vi "DAT Example.vi"() -> ()   [LabVIEW 2013]
panel:
  in  "wavenames (.Vx, etc)":string[](array[string])=["time", "temp", "Bfield", "X0", "Y0", "X1", "Y1", "X2", "Y2", "X3", "Y3", "X4", "Y4", "X5", "Y5"]
  in  "number4":dbl=7.0
  in  "number3":dbl=5.0
  in  "number2":dbl=3.0
  in  "number1":dbl
  out "plot2":cluster{"X":dbl[], "Y":dbl[]}[](graph)
  out "plot1":cluster{"X":dbl[], "Y":dbl[]}[](graph)
  out "plot0":cluster{"X":dbl[], "Y":dbl[]}[](graph)
  in  "Notes":string="date and time are AUTOMATICALLY saved!\nwrite your experiment notes here"
  in  "path":path=path "C:/"
  in  "filename":string="datatest"
  # "- set path to folder\n- set base filename\n   (up to 999,999 files with same base name \n    an be written in one folder)\n- type some comments"
  # "you usually display your data as a XY\ngraphs or charts:"
  # "give everything you are saving a name,\nor else you will become confused!"
  # "combine all of your data using \"build  array\" function\n\nEach entry represents one data point at a partiular time"
  # "\"numbers\" can be\n saved too:"
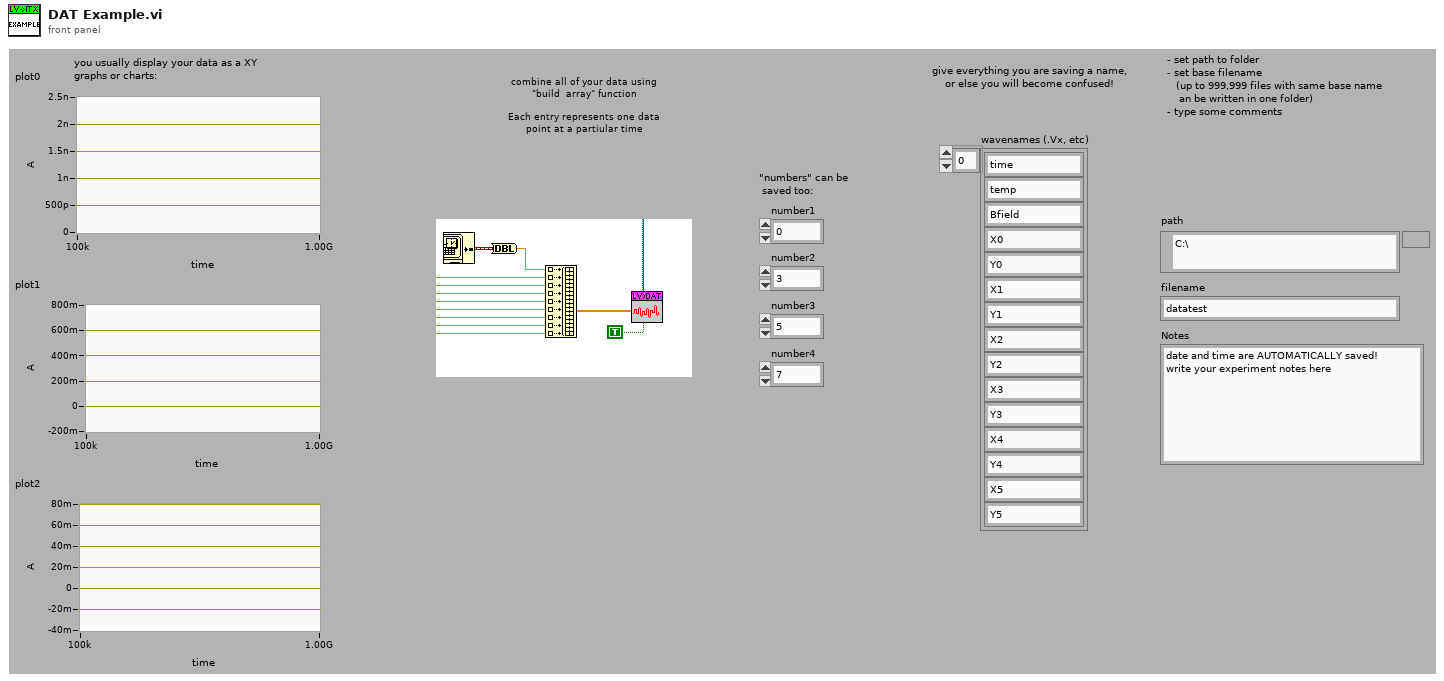
[diagram p1: front panel]
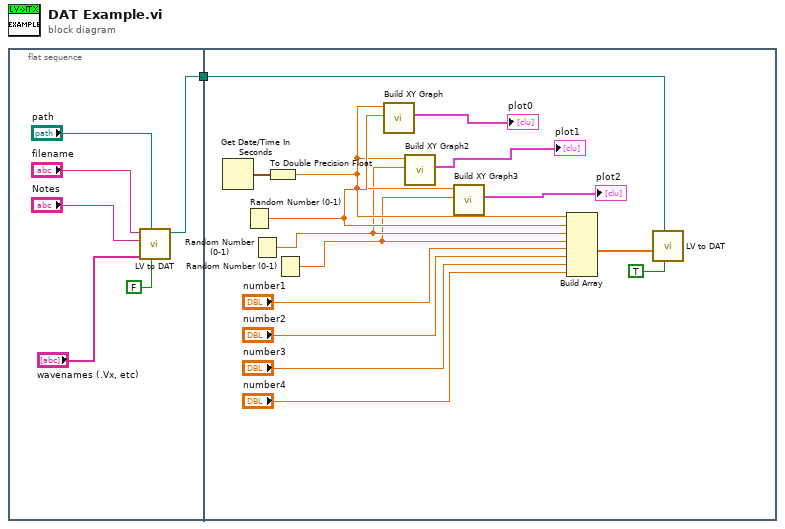
[diagram p0: block diagram]
diagram:
  n1 = flat-sequence {
    tunnel: [w3] -> w1
    tunnel: w1 -> [w21]
    frame #0 {
      n2 = call "LV to DAT.vi"("append to file? (new file:F)"=FALSE, "path"="path", "wavenames (.Vx, etc)"="wavenames (.Vx, etc)", "Comments"="Notes", "filename"="filename") -> ("new file path (Not A Path if cancelled)"=w3:path)  [unwired: 6 in]
    }
    frame #1 {
      n3 = Get Date/Time In Seconds() -> (seconds since 1Jan1904=w15:timestamp)
      n4 = Random Number (0-1)() -> (number: 0 to 1=w14:dbl)
      n5 = Random Number (0-1)() -> (number: 0 to 1=w12:dbl)
      n6 = To Double Precision Float(number=w15) -> (double precision float=w13:dbl)
      n7 = Random Number (0-1)() -> (number: 0 to 1=w11:dbl)
      n8 = call "Build XY Graph"("Y Input"=w14, "X Input"=w13) -> ("XY Graph"=→"plot0":cluster{"X":dbl[], "Y":dbl[]}[])  [unwired: 8 in, 1 out]
      n9 = call "Build XY Graph2"("Y Input"=w12, "X Input"=w13) -> ("XY Graph"=→"plot1":cluster{"X":dbl[], "Y":dbl[]}[])  [unwired: 8 in, 1 out]
      n10 = call "Build XY Graph3"("Y Input"=w11, "X Input"=w13) -> ("XY Graph"=→"plot2":cluster{"X":dbl[], "Y":dbl[]}[])  [unwired: 8 in, 1 out]
      n11 = Build Array(w13, w14, w12, w11, "number1", "number2", "number3", "number4") -> (w16:dbl[])
      n12 = call "LV to DAT.vi"("append to file? (new file:F)"=TRUE, "path"=w21, "Data"=w16) -> ()  [unwired: 8 in, 1 out]
    }
  }
